vi "Load Waveform.vi"(0 "Instrument Handle In":i32, 1 "Ref Channel":i32(ring) caption="Channel" items=["Calc Channel 1", "Calc Channel 2", "Calc Channel 3", "Calc Channel 4", "Ref Channel 1", "Ref Channel 2", "Ref Channel 3", "Ref Channel 4"], 2 "Waveform":dbl[](array[numeric]), 3 "Points":u32, 4 "Count":i32, 5 "error in":errorcluster, 6 "Transfer Type":i32(ring) items=["s8", "s16", "s32", "f32", "f64"], 7 "Voltage Interval":dbl, 8 "Time Interval":dbl, 9 "Voltage Offset":dbl, 10 "Time Offset":dbl, 11 "Type":i32) -> (14 "Instrument Handle Out":i32, 19 "error out":errorcluster)   [LabVIEW 8.6, in "ZTScopeM.lvlib"]
doc: "Load a reference waveform onto the instrument."
uses:
  ZTScopeM.lvlib
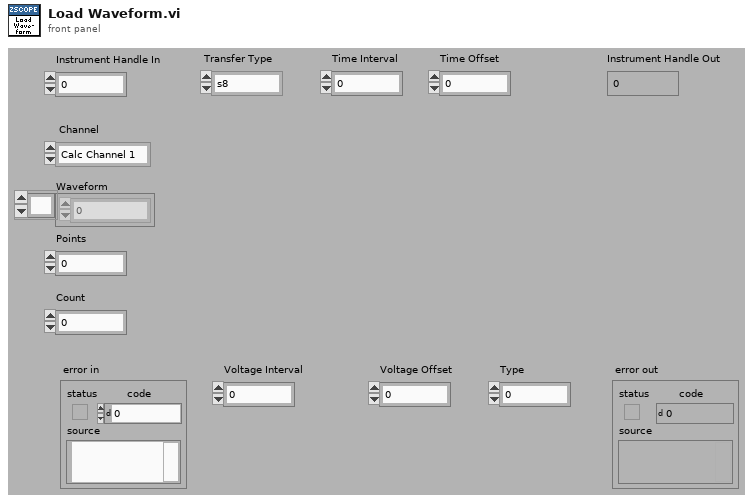
[diagram p1: front panel]
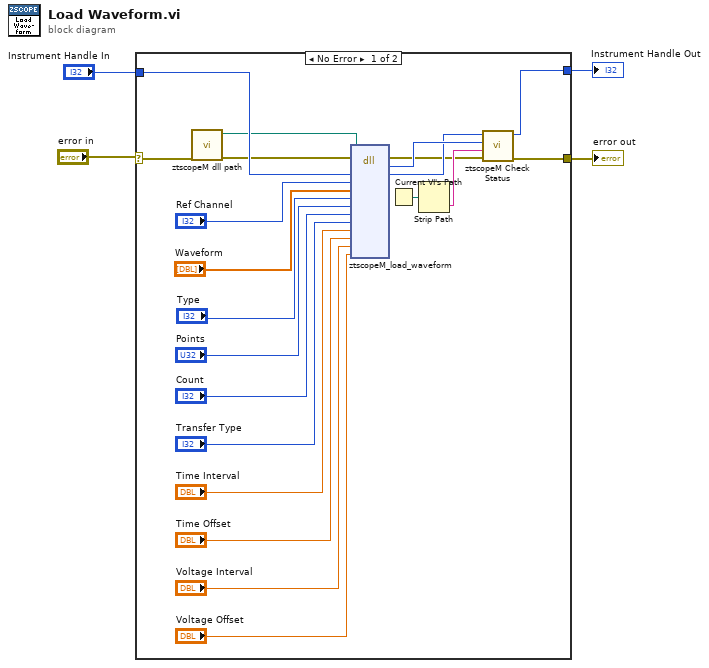
[diagram p0: block diagram]
diagram:
  n1 = case shown="No Error" "error in" {
    selector: "error in" -> [w8 w27]
    tunnel: [w18 w27] -> w1
    tunnel: "Instrument Handle In" -> [w25 w26]
    tunnel: [w17 w26] -> w3
    frame #0 {
      n2 = call "ztscopeM dll path.vi"("error in (no error)"=w8) -> ("error out"=w6:errorcluster, "<instrument>.dll path"=w7:path)  [unwired: 9 in]
      n3 = dll-call lib="C:/Program Files (x86)/National Instruments/LabVIEW 2013/instr.lib/ztscopem/ztscopeM.dll" fn="ztscopeM_load_waveform"(path in=w7, error in=w6, "instrumentHandle"=w25, "referenceChannel"="Ref Channel", "Waveform"="Waveform", "type"="Type", "points"="Points", "count"="Count", "transferType"="Transfer Type", "timeInterval"="Time Interval", "timeOffset"="Time Offset", "voltageInterval"="Voltage Interval", "voltageOffset"="Voltage Offset") -> (error out=w5:errorcluster, w20:i32, "instrumentHandle"=w19:i32)  [unwired: 11 in, 1 out]
      n4 = Current VI's Path() -> (path=w22:path)
      n5 = Strip Path(path=w22) -> (name=w21:string)  [unwired: 1 out]
      n6 = call "ztscopeM Check Status.vi"("error in"=w5, "name of VI"=w21, "status (return code)"=w20, "instrument handle in"=w19) -> ("error out"=w18:errorcluster, "instrument handle out"=w17:i32)  [unwired: 2 in]
    }
    frame #1 {
    }
  }
  "Instrument Handle Out" <- w3
  "error out" <- w1
